vi "Dashboard Main.vi"() -> ()   [LabVIEW 2012]
uses:
  <vilib>/event_ctls.llb/eventvkey.ctl
  <vilib>/Utility/miscctls.llb/LVPointTypeDef.ctl
  <vilib>/Utility/config.llb/Read Key (String).vi
  <vilib>/Utility/config.llb/Read Key (I32).vi
  <vilib>/Utility/config.llb/Write Key (String).vi
  <vilib>/Utility/config.llb/Write Key (I32).vi
  <vilib>/Utility/config.llb/NI_LVConfig.lvlib
panel:
  in  "Camera Settings":T1={"Frate Rate"=30, "Compression"=30, "Size"=0} {"Frate Rate" scale=1.0..30.0; "Size" items=["640x480", "320x240", "160x120"]}
  out "Mode":T2(ring)=enum.""
  out "Camera IP":string="10.16.76.11"
  in  "Dashboard Tab":T3(tab)
  out "Shooter Good":bool
  out "Dashboard Code Verzion":string
  out "Robot Code Verzion":string
  out "Gyro":dbl
  out "Encoder Average":dbl
  out "Right Encoder":dbl
  out "Left Encoder":dbl
  out "Vision Angle":dbl
  in  "Debug Mode":bool
  out "Shooter Good":bool
  out "Shooter Speed":dbl(graph)
  out "Wheel Speed":dbl
  out "Shooter Output":dbl
  out "Shooter Speed":T4(ring)
  out "Robot IP":string="0.0.0.0"
  out "MotorSlide4":dbl(slide) scale=-1.0..1.0 scale format="%#_2e"
  out "MotorSlide3":dbl(slide) scale=-1.0..1.0 scale format="%#_2e"
  out "MotorSlide2":dbl(slide) scale=-1.0..1.0 scale format="%#_2e"
  in  "MotorName3":string="Front Left"
  in  "MotorName4":string="Front Right"
  in  "MotorName1":string="Rear Left"
  in  "MotorName2":string="Rear Right"
  out "MotorChart4":dbl(graph)
  out "MotorChart3":dbl(graph)
  out "MotorChart2":dbl(graph)
  out "MotorSlide1":dbl(slide) scale=-1.0..1.0 scale format="%#_2e"
  out "MotorChart1":dbl(graph)
  out "JS1 Z":dbl(slide) scale=-1.0..1.0 scale format="%#_2e"
  out "JS2 Z":dbl(slide) scale=-1.0..1.0 scale format="%#_2e"
  out "Joystick 1":cluster{"X":dbl, "Y":dbl}[](graph)
  out "Joystick 2":cluster{"X":dbl, "Y":dbl}[](graph)
  out "JS Buttons 1":T5
  out "JS Buttons 2":T5
  out "Battery Value":dbl(slide) scale=0.0..14.0 scale format="%#_2e"
  out "Battery":sgl(graph)
  in  "Slider":dbl(slide) scale=0.0..100.0 scale format="%#_3g"
  in  "On/Off":bool caption="Solenoid"
  in  "Test Name":u16(ring) items=["Select the test to run...", "Example Test", "-------------------------------", "List of tests is built in robot code.", "Replace with your own automated tests."]
  in  "Test Tree":string(tree)
  in  "Motor":cluster{"Value":dbl, "Enable":bool} {"Value" scale=-1.0..1.0 scale format="%#_3g"}
  out "Progress":T6 {"Test Progress" scale=0.0..100.0}
  in  "Rev/Fwd":cluster{"Forward":bool, "Reverse":bool}
  in  "Ring":u16(ring) items=["Auto", "Fixed indoor", "Fixed outdoor 1", "Fixed outdoor 2", "Fixed fluorescent 1", "Fixed fluorescent 2", "Hold current"]
  in  "Listbox":i32(listbox)
  in  "Viewer":T7(tab)
  out "Mbps":dbl format="%#.1g"
  in  "Enable":bool=TRUE
  in  "DB Camera Config":bool
  out "Mbps":bool
  out "fps":dbl format="%#.1g"
  out "Image Error Message":string="Timeout in Camera Communications"
  out "Camera Image":T8(plugin-control)
  out "Buttons 1":cluster{"1":bool, "2":bool, "3":bool}
  out "Kinect 1":cluster{"X":dbl, "Y":dbl, "Z":dbl} {"X" scale=1.0..-1.0; "Y" scale=1.0..-1.0; "Z" scale=1.0..-1.0}
  out "Buttons 2":cluster{"1":bool, "2":bool, "3":bool}
  out "Kinect 2":cluster{"X":dbl, "Y":dbl, "Z":dbl} {"X" scale=1.0..-1.0; "Y" scale=1.0..-1.0; "Z" scale=1.0..-1.0}
  out "Version":string
  out "Skeleton Picture":picture
  out "Players":i8
  out "Tree":string(tree)
  # "Old Info"
  # "Drive & Motors"
  # "Robot IP:"
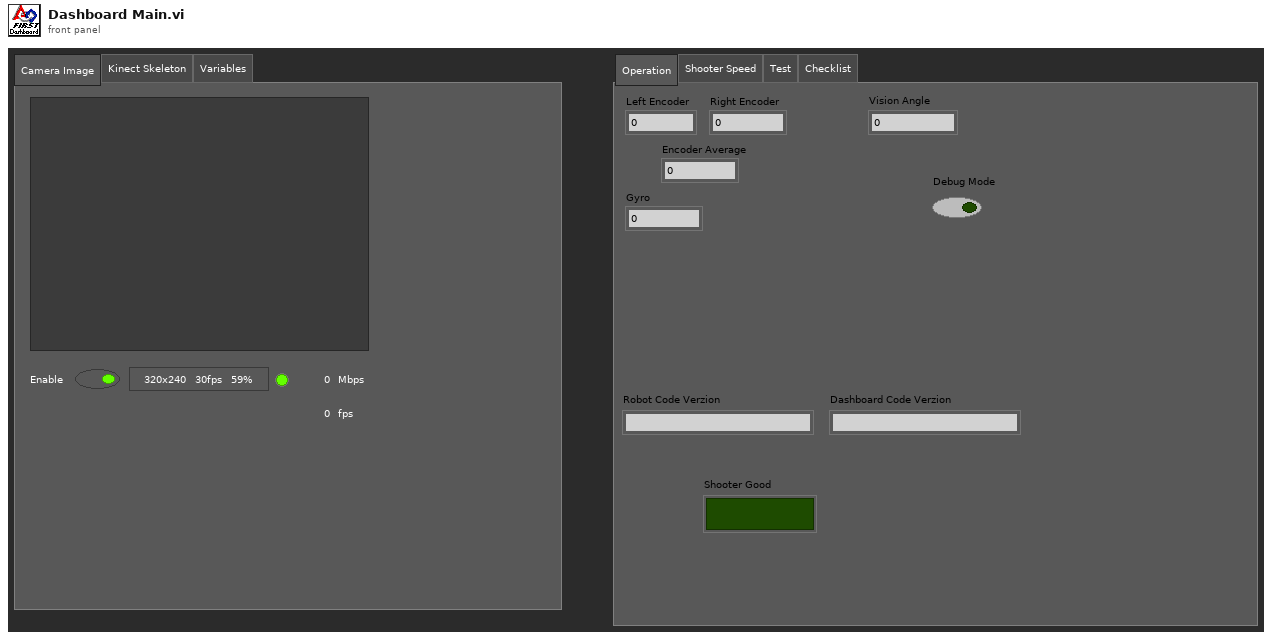
[diagram p1: front panel]
types:
  T1 = cluster{"Frate Rate":i32, "Compression":i32, "Size":u16}
  T2 = enum8{"Tele-Op Disabled", "Tele-Op Enabled", "Auto Disabled", "Auto Enabled", "Test Disabled", "Test Enabled", ""}
  T3 = enum32{"Operation", "Shooter Speed", "Test", "Checklist"}
  T4 = enum16{"Off", "Close Pyramid 3pt", "Far Pyramid 3pt", "Feeder Shot"}
  T5 = cluster{bool, bool, bool, bool, bool, bool, bool, bool, bool, bool, bool, bool}
  T6 = cluster{"Test Progress":u8, "Test Progress Text":string}
  T7 = enum32{"Camera Image", "Kinect Skeleton", "Variables"}
  T8 = typedef "IMAQ Image.ctl" = refnum<image>
  T9 = typedef "Image Type" = u32
  T10 = cluster{"Competition mode":bool, "Robot Link":bool, "Autonomous":bool, "Enabled":bool, "E-Stop":bool, "Simulated":bool, "TestMode":bool, "Docked Window":bool}
  T11 = cluster{"Boolean Array[0]":bool, "Boolean Array[1]":bool, "Boolean Array[2]":bool, "Boolean Array[3]":bool, "Boolean Array[4]":bool, "Boolean Array[5]":bool, "Boolean Array[6]":bool, "Boolean Array[7]":bool, "Boolean Array[8]":bool, "Boolean Array[9]":bool, "Boolean Array[10]":bool, "Boolean Array[11]":bool}
  T12 = typedef "LVPointTypeDef.ctl" = cluster{"Horizontal":i16, "Vertical":i16}
  T13 = typedef "LVRectTypeDef.ctl" = cluster{"Left":i16, "Top":i16, "Right":i16, "Bottom":i16}
  T14 = typedef "LVBoundsTypeDef.ctl" = cluster{"Width":u32, "Height":u32}
  T15 = typedef "SkeletonTrackState.ctl" = enum32{"NotTracked", "PositionOnly", "Tracked"}
  T16 = cluster{"TrackingState":u8[], "Position":cluster{"x":sgl, "y":sgl, "z":sgl}, cluster{"x":sgl, "y":sgl, "z":sgl, sgl}[], "TrackState":T15}
  T17 = cluster{cluster{"ScaledToPercentRange":dbl, "ScaledToPercentRange":dbl, "ScaledToPercentRange":dbl}, cluster{bool, bool, bool}}[]
  T18 = cluster{cluster{"ScaledToPercentRange":dbl, "ScaledToPercentRange":dbl, "ScaledToPercentRange":dbl}, cluster{bool, bool, bool}}
  T19 = cluster{"ScaledToPercentRange":dbl, "ScaledToPercentRange":dbl, "ScaledToPercentRange":dbl}
  T20 = typedef "NI_LVConfig.lvlib/Config Data RefNum.ctl" = refnum<k1>
  T21 = typedef "eventvkey.ctl" = enum16{"ASCII", "Enter", "Return", "Shift", "Ctrl", "Alt", "Cmd", "Opt", "Caps", "NumLock", "Clear", "Break", "Up", "Down", "Left", "Right", "Insert", "Delete", "Home", "End", "PageUp", "PageDown", "Escape", "Help", "Pause", "ScrollLock", "F1", "F2", "F3", "F4", "F5", "F6", "F7", "F8", "F9", "F10", "F11", "F12", "F13", "F14", "F15", "F16", "F17", "F18", "F19", "F20", "F21", "F22", "F23", "F24", "Play", "VolumeUp", "VolumeDown", "Mute", "Two Byte Char"}
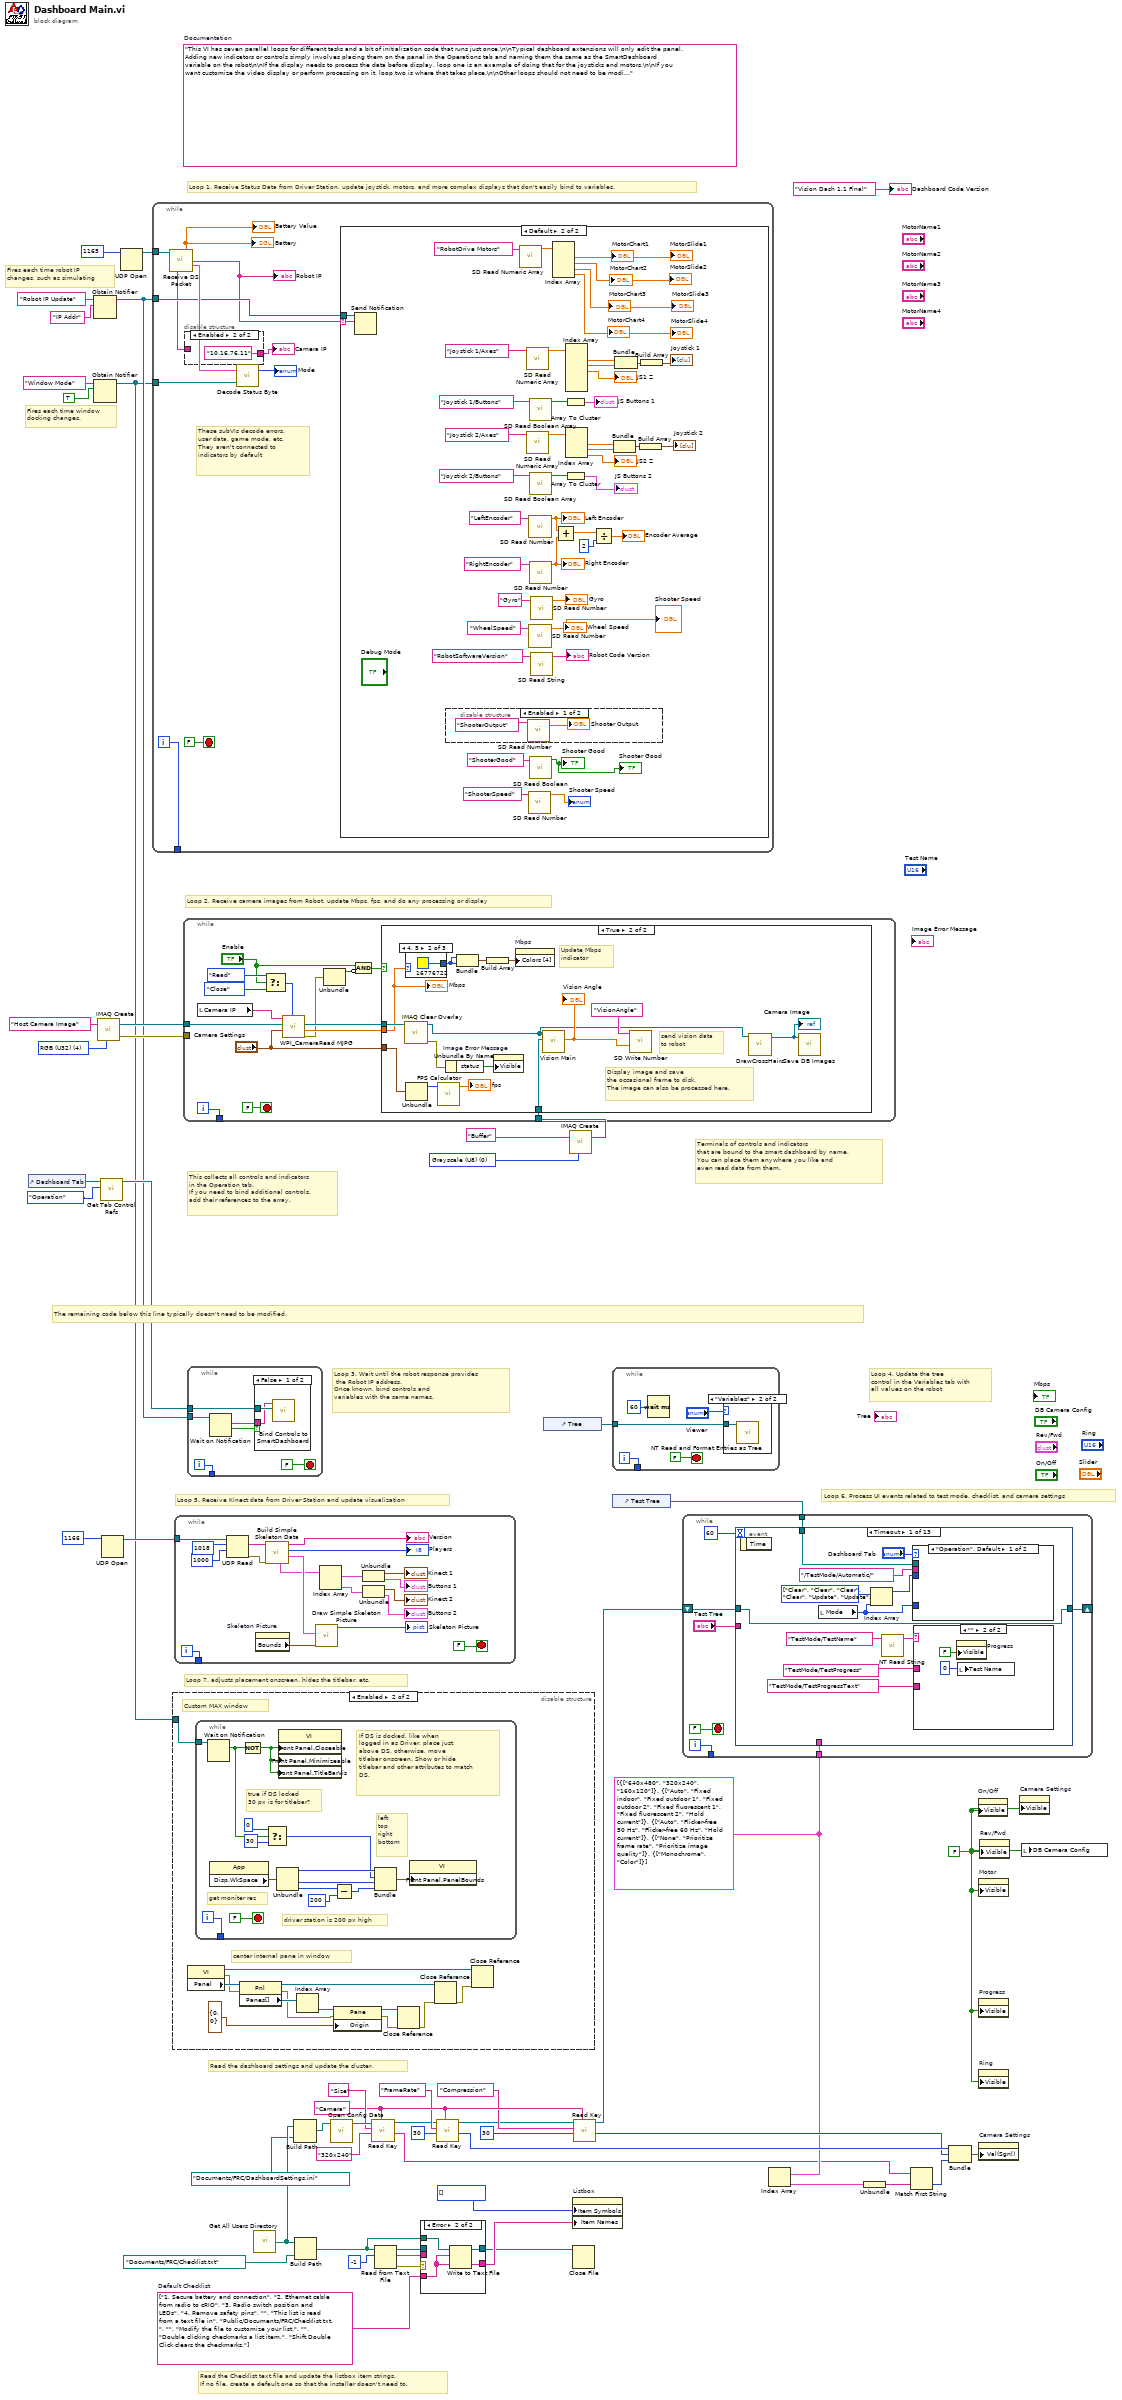
[diagram p0: block diagram]
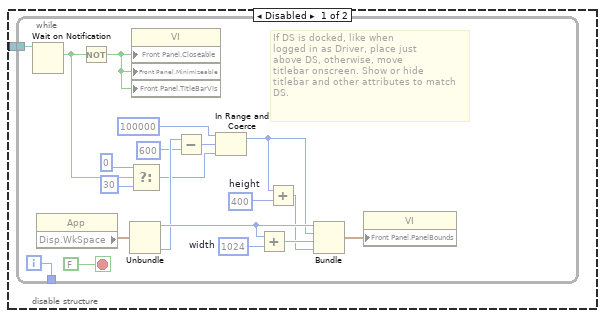
[diagram p2: hidden frame]
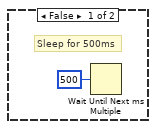
[diagram p4: hidden frame]
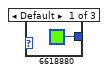
[diagram p5: hidden frame]
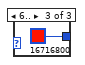
[diagram p6: hidden frame]
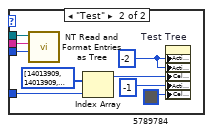
[diagram p8: hidden frame]
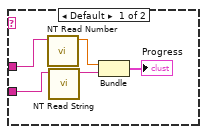
[diagram p9: hidden frame]
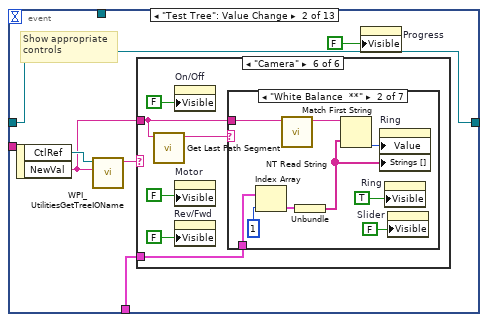
[diagram p10: hidden frame]
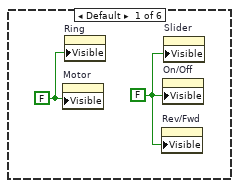
[diagram p11: hidden frame]
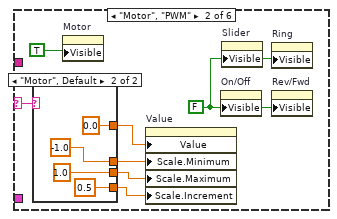
[diagram p12: hidden frame]
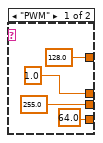
[diagram p13: hidden frame]
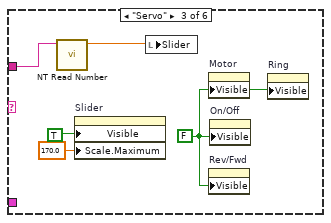
[diagram p14: hidden frame]
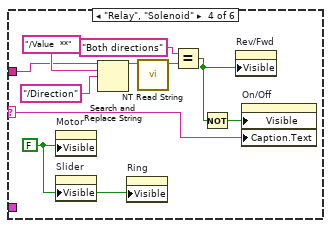
[diagram p15: hidden frame]
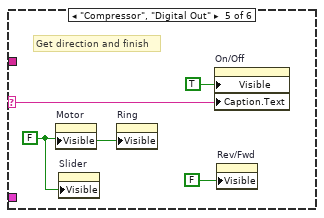
[diagram p16: hidden frame]
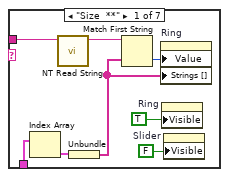
[diagram p17: hidden frame]
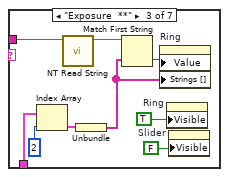
[diagram p18: hidden frame]
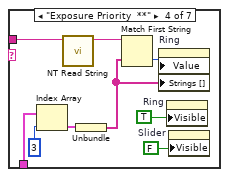
[diagram p19: hidden frame]
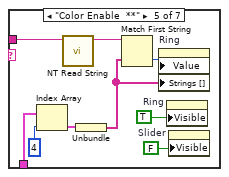
[diagram p20: hidden frame]
diagram:
  w3 = T9 0 items=["Grayscale (U8)", "Grayscale (I16)", "Grayscale (SGL)", "Complex (CSG)", "RGB (U32)", "HSL (U32)", "RGB (U64)", "Grayscale (U16)"] ("Image Type")
  w25 = "Camera"
  w17 = cluster{string[]}[] [{["640x480", "320x240", "160x120"]}, {["Auto", "Fixed indoor", "Fixed outdoor 1", "Fixed outdoor 2", "Fixed fluorescent 1", "Fixed fluorescent 2", "Hold current"]}, {["Auto", "Flicker-free 50 Hz", "Flicker-free 60 Hz", "Hold current"]}, {["None", "Prioritize frame rate", "Prioritize image quality"]}, {["Monochrome", "Color"]}]
  w33 = string[] ["1. Secure battery and connection", "2. Ethernet cable from radio to cRIO", "3. Radio switch position and LEDs", "4. Remove safety pins", "", "This list is read from a text file in", "Public/Documents/FRC/Checklist.txt.", "", "Modify the file to customize your list.", "", "Double clicking checkmarks a list item.", "Shift Double Click clears the checkmarks."]  # Default Checklist
  w31 = FALSE ("Visible")
  (unwired) "This VI has seven parallel loops for different tasks and a bit of initialization code that runs just once.\n\nTypical dashboard extensions will only edit the panel. Adding new indicators or controls simply involves placing them on the panel in the Operations tab and naming them the same as the SmartDashboard variable on the robot\n\nIf the display needs to process the data before display, loop one is an example of doing that for the joysticks and motors.\n\nIf you want customize the video display or perform processing on it, loop two is where that takes place.\n\nOther loops should not need to be modified. They are pretty standard, and document the task they perform."  # Documentation
  w54 = T9 4 items=["Grayscale (U8)", "Grayscale (I16)", "Grayscale (SGL)", "Complex (CSG)", "RGB (U32)", "HSL (U32)", "RGB (U64)"] ("Image Type")
  # "Fires each time robot IP\nchanges, such as simulating"
  # "Fires each time window\ndocking changes."
  # "Read the Checklist text file and update the listbox item strings.\nIf no file, create a default one so that the installer doesn't need to."
  # "This collects all controls and indicators\nin the Operation tab.\nIf you need to bind additional controls,\nadd their references to the array."
  # "The remaining code below this line typically doesn't need to be modified."
  # "Loop 6. Process UI events related to test mode, checklist, and camera settings"
  # "Read the dashboard settings and update the cluster."
  # "Terminals of controls and indicators\nthat are bound to the smart dashboard by name.\nYou can place them anywhere you like and\neven read data from them."
  # "Loop 4. Update the tree\ncontrol in the Variables tab with\nall values on the robot"
  # "Loop 3. Wait until the robot response provides\n the Robot IP address.\nOnce known, bind controls and\nvariables with the same names."
  # "Loop 5. Receive Kinect data from Driver Station and update visualization"
  # "Loop 7. adjusts placement onscreen, hides the titlebar, etc."
  # "Loop 1. Receive Status Data from Driver Station, update joystick, motors, and more complex displays that don't easily bind to variables."
  # "Loop 2. Receive camera images from Robot, update Mbps, fps, and do any processing or display"
  n1 = control-ref of="Dashboard Tab"() -> (w47:refnum<vi>)
  n2 = Obtain Notifier(name (unnamed)="Robot IP Update", notification data type="IP Addr" ("name (unnamed)")) -> (notifier out=w44:refnum<notifier>)  [unwired: 2 in, 2 out]
  n3 = Obtain Notifier(name (unnamed)="Window Mode", notification data type=TRUE) -> (notifier out=w37:refnum<notifier>)  [unwired: 2 in, 2 out]
  n4 = call "IMAQ Create"("Image Name"="Host Camera Image", "Image Type"=w54) -> ("New Image"=w52:T8, "error out"=w51:errorcluster)  [unwired: 2 in, 1 out]
  n5 = call <vilib>:"Get Tab Control Refs.vi"("Page Index"=enum32{"Operation", "Test"}."Operation" ("Dashboard Tab"), "TabControl in"=w47) -> ("ControlsOnPage"=w48:refnum<vi>[])  [unwired: 9 in]
  n6 = UDP Open(11:u16 1166 ("port")) -> (port=w49:refnum<k16>)  [unwired: 2 in, 4 out]
  n7 = UDP Open(11:u16 1165 ("port")) -> (port=w55:refnum<k16>)  [unwired: 2 in, 4 out]
  n8 = while {
    tunnel: w55 -> [w65]
    tunnel: w44 -> [w60]
    tunnel: w37 -> [w63]
    tunnel: [w61] -> _
    i -> [w61]
    stop <- FALSE stop-if-true
    # "These subVIs decode errors, user data, game mode, etc.\nThey aren't connected to indicators by default"
    n9 = call "Receive DS Packet.vi"("Recv Socket"=w65) -> ("Battery"=→"Battery" →"Battery Value":sgl, "Robot IP Address"=w59:string, "Status"=w66:T10, "Camera IP Address"=w57:string)  [unwired: 1 in, 10 out]
    "Robot IP" <- w59
    n10 = disable-structure shown="Enabled" {
      disable-tunnel: [w68 "10.16.76.11" ("Camera IP")] -> w58
      disable-tunnel: w57 -> [w68 _]
      frame Disabled {
      }
      frame Enabled {
      }
    }
    "Camera IP" <- w58
    n11 = call "Decode Status Byte.vi"("Window Mode Notifier"=w63, "Status"=w66) -> ("Mode"=→"Mode":T2)  [unwired: 1 out]
    n12 = case shown="Default" w59 {
      selector: w59 -> [_ w87]
      tunnel: w60 -> [_ w88]
      frame "0.0.0.0" {
        # "Robot not responding, don't poll the variables"
      }
      frame Default {
        n13 = Send Notification(notification=w87, notifier=w88) -> ()  [unwired: 1 in, 2 out]
        n14 = disable-structure shown="Enabled" {
          frame Enabled {
            n15 = call <vilib>:"SD Read Number.vi"("Name"="ShooterOutput") -> ("Numeric"=→"Shooter Output":dbl)  [unwired: 8 in, 2 out]
          }
          frame Disabled {
          }
        }
        n16 = call <vilib>:"SD Read Numeric Array.vi"("Name"="RobotDrive Motors") -> ("Numeric Array"=w111:dbl[])  [unwired: 8 in, 2 out]
        n17 = call <vilib>:"SD Read Numeric Array.vi"("Name"="Joystick 1/Axes") -> ("Numeric Array"=w104:dbl[])  [unwired: 8 in, 2 out]
        n18 = call <vilib>:"SD Read Numeric Array.vi"("Name"="Joystick 2/Axes") -> ("Numeric Array"=w98:dbl[])  [unwired: 8 in, 2 out]
        n19 = call <vilib>:"SD Read Number.vi"("Name"="ShooterSpeed") -> ("Numeric"=→"Shooter Speed":dbl)  [unwired: 8 in, 2 out]
        n20 = call <vilib>:"SD Read Number.vi"("Name"="LeftEncoder") -> ("Numeric"=w83:dbl)  [unwired: 8 in, 2 out]
        "Left Encoder" <- w83
        n21 = call <vilib>:"SD Read Number.vi"("Name"="WheelSpeed") -> ("Numeric"=→"Wheel Speed" →"Shooter Speed":dbl)  [unwired: 8 in, 2 out]
        n22 = call <vilib>:"SD Read Boolean Array.vi"("Name"="Joystick 1/Buttons") -> ("Boolean Array"=w106:bool[])  [unwired: 8 in, 2 out]
        n23 = call <vilib>:"SD Read Boolean Array.vi"("Name"="Joystick 2/Buttons") -> ("Boolean Array"=w97:bool[])  [unwired: 8 in, 2 out]
        n24 = call <vilib>:"SD Read Number.vi"("Name"="RightEncoder") -> ("Numeric"=w82:dbl)  [unwired: 8 in, 2 out]
        "Right Encoder" <- w82
        n25 = call <vilib>:"SD Read Boolean.vi"("Name"="ShooterGood") -> ("Boolean"=→"Shooter Good" →"Shooter Good":bool)  [unwired: 8 in, 2 out]
        n26 = call <vilib>:"SD Read Number.vi"("Name"="Gyro") -> ("Numeric"=→"Gyro":dbl)  [unwired: 8 in, 2 out]
        n27 = call <vilib>:"SD Read String.vi"("Name"="RobotSoftwareVersion") -> ("String"=→"Robot Code Verzion":string)  [unwired: 8 in, 2 out]
        n28 = Index Array(array=w111) -> (element #1=→"MotorChart1" →"MotorSlide1":dbl, element #2=→"MotorSlide2" →"MotorChart2":dbl, element #3=→"MotorChart3" →"MotorSlide3":dbl, element #4=→"MotorChart4" →"MotorSlide4":dbl)  [unwired: 4 in]
        n29 = Add(x=w83, y=w82) -> (x+y=w80:dbl)
        n30 = Array To Cluster(array=w106) -> (cluster=→"JS Buttons 1":T11)
        n31 = Array To Cluster(array=w97) -> (cluster=→"JS Buttons 2":T11)
        n32 = Index Array(array=w104) -> (element #1=w101:dbl, element #2=w102:dbl, element #3=→"JS1 Z":dbl)  [unwired: 6 in, 3 out]
        n33 = Index Array(array=w98) -> (element #1=w93:dbl, element #2=w92:dbl, element #3=→"JS2 Z":dbl)  [unwired: 3 in]
        n34 = Divide(x=w80, y=2) -> (x/y=→"Encoder Average":dbl)
        n35 = Bundle("Numeric"=w93, "Numeric"=w92) -> (w94:cluster{"Numeric":dbl, "Numeric":dbl})  [unwired: 1 in]
        n36 = Bundle("Numeric"=w101, "Numeric"=w102) -> (w100:cluster{"Numeric":dbl, "Numeric":dbl})  [unwired: 1 in]
        n37 = Build Array(w94) -> (→"Joystick 2":cluster{"Numeric":dbl, "Numeric":dbl}[])
        n38 = Build Array(w100) -> (→"Joystick 1":cluster{"Numeric":dbl, "Numeric":dbl}[])
      }
    }
  }
  n39 = disable-structure shown="Enabled" {
    disable-tunnel: w37 -> [w117 w150]
    frame Disabled {
      n40 = while {
        tunnel: w117 -> [w136]
        tunnel: [w134] -> _
        i -> [w134]
        stop <- FALSE stop-if-true
        w126 = 1024  # width
        w129 = 400  # height
        # "If DS is docked, like when\nlogged in as Driver, place just\nabove DS, otherwise, move\ntitlebar onscreen. Show or hide\ntitlebar and other attributes to match\nDS."
        n41 = Wait on Notification(notifier=w136) -> (notification=w121:bool)  [unwired: 3 in, 3 out]
        n42 = property class="App"() -> ("Disp.WkSpace"=w132:T13)  [unwired: 2 in, 2 out]
        n43 = Not(x=w121) -> (.not. x?=w135:bool)
        n44 = Unbundle(w132) -> ("Left"=w130:i16, "Bottom"=w127:i16)  [unwired: 2 out]
        n45 = Select(t=0, s=w121, f=30) -> (s? t:f=w120:i32)
        n46 = property class="VI"("Front Panel.Closeable"=w135, "Front Panel.Minimizeable"=w135, "Front Panel.TitleBarVis"=w135) -> ()  [unwired: 2 in, 2 out]
        n47 = Subtract(x=w127, y=600) -> (x-y=w124:i32)
        n48 = In Range and Coerce(upper limit=100000, x=w124, lower limit=w120) -> (coerced(x)=w118:i32)  [unwired: 1 out]
        n49 = Add(x=w130, y=w126) -> (x+y=w131:i32)
        n50 = Add(x=w118, y=w129) -> (x+y=w128:i32)
        n51 = Bundle("Left"=w130, w118, w131, w128) -> (w133:cluster{"Left":i16, i32, i32, i32})  [unwired: 1 out]
        n52 = property class="VI"("Front Panel.PanelBounds"=w133) -> ()  [unwired: 2 in, 2 out]
      }
    }
    frame Enabled {
      # "center internal pane in window"
      # "Custom MAX window"
      n53 = property class="VI"() -> (reference out=w143:refnum<vi>, error out=w142:errorcluster, "Panel"=w149:refnum<vi>)  [unwired: 2 in]
      n54 = while {
        tunnel: w150 -> [w164]
        tunnel: [w162] -> _
        i -> [w162]
        stop <- FALSE stop-if-true
        # "driver station is 200 px high"
        # "true if DS locked\n30 px is for titlebar?"
        # "left\ntop\nright\nbottom"
        # "get moniter rez"
        # "If DS is docked, like when\nlogged in as Driver, place just\nabove DS, otherwise, move\ntitlebar onscreen. Show or hide\ntitlebar and other attributes to match\nDS."
        n55 = Wait on Notification(notifier=w164) -> (notification=w156:bool)  [unwired: 3 in, 3 out]
        n56 = property class="App"() -> ("Disp.WkSpace"=w160:T13)  [unwired: 2 in, 2 out]
        n57 = Not(x=w156) -> (.not. x?=w163:bool)
        n58 = Select(t=0, s=w156, f=30) -> (s? t:f=w154:i32)
        n59 = Unbundle(w160) -> ("Left"=w159:i16, "Right"=w155:i16, "Bottom"=w152:i16)  [unwired: 1 out]
        n60 = property class="VI"("Front Panel.Closeable"=w163, "Front Panel.Minimizeable"=w163, "Front Panel.TitleBarVis"=w163) -> ()  [unwired: 2 in, 2 out]
        n61 = Subtract(x=w152, y=i16 200) -> (x-y=w153:i16)
        n62 = Bundle("Left"=w159, w154, "Right"=w155, w153) -> (w161:cluster{"Left":i16, i32, "Right":i16, i16})  [unwired: 1 out]
        n63 = property class="VI"("Front Panel.PanelBounds"=w161) -> ()  [unwired: 2 in, 2 out]
      }
      n64 = property class="Pnl"(reference=w149, error in=w142) -> (reference out=w144:refnum<vi>, error out=w141:errorcluster, "Panes[]"=w148:refnum<vi>[])
      n65 = Index Array(array=w148) -> (element=w147:refnum<vi>)  [unwired: 1 in]
      n66 = property class="Pane"(reference=w147, error in=w141, "Origin"=T12 {"Horizontal"=0, "Vertical"=0}) -> (reference out=w145:refnum<vi>, error out=w140:errorcluster)
      n67 = Close Reference(reference=w145, error in (no error)=w140) -> (error out=w139:errorcluster)
      n68 = Close Reference(reference=w144, error in (no error)=w139) -> (error out=w138:errorcluster)
      n69 = Close Reference(reference=w143, error in (no error)=w138) -> ()  [unwired: 1 out]
    }
  }
  n70 = while {
    tunnel: w49 -> [w182]
    tunnel: [w167] -> _
    i -> [w167]
    stop <- FALSE stop-if-true
    n71 = UDP Read(connection ID=w182, max size (548)=1018 ("bytes to read"), timeout ms (25000)=1000) -> (data out=w176:string, error out=w166:errorcluster)  [unwired: 1 in, 3 out]
    n72 = property on="Skeleton Picture" class="Pict"() -> ("Bounds"=w178:T14)  [unwired: 2 in, 2 out]
    n73 = call "Build Simple Skeleton Data.vi"("error in (no error)"=w166, "data in"=w176) -> ("Skeleton Data"=w177:T16, "NumPlayers"=→"Players":i8, "Version String"=→"Version":string, "Simple Joystick Info"=w174:T17)  [unwired: 5 in, 1 out]
    n74 = call "Draw Simple Skeleton Picture.vi"("Bounds"=w178, "Simple Skeleton"=w177) -> ("new picture out"=→"Skeleton Picture":picture)  [unwired: 9 in]
    n75 = Index Array(array=w174) -> (element #1=w173:T18, element #2=w172:T18)  [unwired: 2 in]
    n76 = Unbundle(w173) -> (→"Kinect 1":T19, →"Buttons 1":cluster{bool, bool, bool})
    n77 = Unbundle(w172) -> (→"Kinect 2":T19, →"Buttons 2":cluster{bool, bool, bool})
  }
  n78 = while {
    tunnel: w48 -> [w190]
    tunnel: w44 -> [w187]
    tunnel: [w185] -> _
    i -> [w185]
    stop <- FALSE stop-if-true
    n79 = Wait on Notification(notifier=w187) -> (notification=w186:string, timed out?=w188:bool)  [unwired: 3 in, 2 out]
    n80 = case shown="False" w188 {
      tunnel: w190 -> [w192 _]
      tunnel: w186 -> [w191 _]
      frame False {
        n81 = call <vilib>:"Bind Controls to SmartDashboard.vi"("Bound Control Refs"=w192, "Server IP Address"=w191) -> ()  [unwired: 10 in]
      }
      frame True {
      }
    }
  }
  n82 = call "Get All Users Directory.vi"() -> ("All User Path"=w30:path)
  n83 = Build Path(base path=w30, name or relative path=path "Documents/FRC/DashboardSettings.ini") -> (appended path=w29:path)
  n84 = Build Path(base path=w30, name or relative path=path "Documents/FRC/Checklist.txt") -> (appended path=w34:path)
  n85 = call <vilib>:"Open Config Data.vi"("configuration file path"=w29) -> ("refnum"=w28:T20)  [unwired: 8 in, 2 out]
  n86 = call-poly <vilib>:"Read Key.vi"("section"=w25, "default value"="320x240", "key"="Size", "refnum"=w28) -> ("value"=w15:string, "refnum out"=w10:T20)  [unwired: 2 in, 4 out]
  n87 = Read from Text File(file (use dialog)=w34, count=-1 ("timeout ms (25000)")) -> (refnum out=w12:refnum<file>, text=w35:string[], error out=w36:errorcluster)  [unwired: 2 in, 1 out]
  n88 = case shown="Error" w36 {
    tunnel: w35 -> [w194 _]
    tunnel: [w194 w196] -> w32
    tunnel: w33 -> [_ w196]
    tunnel: w34 -> [_ w197]
    tunnel: [w193 w195] -> w11
    tunnel: w12 -> [w193 _]
    frame No Error {
    }
    frame Error {
      n89 = Write to Text File(file (use dialog)=w197, text=w196) -> (refnum out=w195:refnum<file>)  [unwired: 2 in, 2 out]
    }
  }
  n90 = call-poly <vilib>:"Read Key.vi"("section"=w25, "default value"=30, "key"="FrameRate", "refnum"=w10) -> ("value"=w20:i32, "refnum out"=w9:T20)  [unwired: 1 in, 5 out]
  n91 = control-ref of="Tree"() -> (w6:refnum<vi>)
  n92 = call "IMAQ Create"("Image Name"="Buffer", "Image Type"=w3) -> ("New Image"=w2:T8)  [unwired: 3 in, 1 out]
  n93 = while {
    tunnel: w52 -> [w208]
    tunnel: w51 -> [_]
    tunnel: [w211] -> _
    tunnel: w2 -> [w198]
    i -> [w211]
    stop <- FALSE stop-if-true
    n94 = local read "Camera IP"() -> (w210:string)
    n95 = Select(t=enum16{"Read", "Reopen", "Close"}."Read" ("Operation"), s="Enable", f=enum16{"Read", "Reopen", "Close"}."Close" ("Operation")) -> (s? t:f=w203:enum16{"Read", "Reopen", "Close"})
    n96 = call <vilib>:"WPI_CameraRead MJPG.vi"("Operation"=w203, "Camera Settings"="Camera Settings", "Image"=w208, "address"=w210) -> ("error out"=w202:errorcluster, "Bandwidth (kbps)"=w206:dbl, "Image Out"=w207:T8)  [unwired: 5 in]
    n97 = Unbundle(w202) -> ("status"=w200:bool)  [unwired: 2 out]
    n98 = Compound Arithmetic op=AND("Enable", invert w200) -> (w199:bool)
    n99 = case shown="True" w199 {
      tunnel: "Camera Settings" -> [_ w220]
      tunnel: w207 -> [_ w223]
      tunnel: w206 -> [_ w222]
      tunnel: w198 -> [_ w218]
      frame False {
        # "Sleep for 500ms"
        n100 = Wait Until Next ms Multiple(millisecond multiple=u32 500) -> ()  [unwired: 1 out]
      }
      frame True {
        # "send vision data\nto robot"
        # "Display image and save\nthe occasional frame to disk.\nThe image can also be processed here."
        # "Update Mbps\nindicator"
        n101 = call "IMAQ Clear Overlay"("Image"=w223) -> ("error out"=w227:errorcluster, "Image Out"=w214:T8)  [unwired: 2 in, 7 out]
        n102 = case shown="4, 5" w222 {
          tunnel: [u32 6618880 ("Color Box") u32 16776722 ("Color Box") u32 16716800 ("Color Box")] -> w224
          frame Default {
          }
          frame 4, 5 {
          }
          frame 6.. {
          }
        }
        n103 = Unbundle(w220) -> ("Frate Rate"=w219:i32)  [unwired: 2 out]
        n104 = call "FPS Calculator.vi"("Average Count"=w219) -> ("fps"=→"fps":dbl)  [unwired: 10 in]
        n105 = Unbundle By Name(w227) -> ("status"=w228:bool)
        n106 = Bundle("Color Box"=w224, "Color Box"=w224) -> (w226:cluster{"Color Box":u32, "Color Box":u32})  [unwired: 1 out]
        n107 = Build Array(w226) -> (w225:cluster{"Color Box":u32, "Color Box":u32}[])
        n108 = property on="Image Error Message" class="Str"("Visible"=w228) -> ()  [unwired: 2 in, 2 out]
        n109 = property on="Mbps" class="Bool (strict)"("Colors [4]"=w225) -> ()  [unwired: 2 in, 2 out]
        n110 = call "Vision Main.vi"("Frame Buffer"=w218, "Camera Image"=w214) -> ("Chosen Target Angle"=w216:dbl)  [unwired: 8 in, 1 out]
        "Vision Angle" <- w216
        n111 = call <vilib>:"SD Write Number.vi"("Numeric"=w216, "Name"="VisionAngle") -> ()  [unwired: 8 in, 2 out]
        n112 = call "DrawCrossHairs.vi"("Image In"=w214) -> ("Image Out"=w215:T8)  [unwired: 10 in]
        "Camera Image" <- w215
        n113 = call "Save DB Images.vi"("Image"=w215) -> ()  [unwired: 2 in, 1 out]
        "Mbps" <- w222
      }
    }
  }
  n114 = property on="Listbox" class="LstBox (strict)"("Item Symbols"=i32[] [], "Item Names"=w32) -> ()  [unwired: 2 in, 2 out]
  n115 = Close File(refnum=w11) -> ()  [unwired: 1 in, 2 out]
  n116 = call-poly <vilib>:"Read Key.vi"("section"=w25, "default value"=30, "key"="Compression", "refnum"=w9) -> ("value"=w19:i32, "refnum out"=w7:T20)  [unwired: 1 in, 5 out]
  n117 = while {
    tunnel: [w233] -> _
    tunnel: w6 -> [w232]
    i -> [w233]
    stop <- FALSE stop-if-true
    n118 = Wait (ms)(milliseconds to wait=u32 60) -> ()  [unwired: 1 out]
    n119 = case shown="\"Variables\"" "Viewer" {
      tunnel: w232 -> [_ w237]
      frame Default {
      }
      frame "Variables" {
        n120 = call <vilib>:"NT Read and Format Entries as Tree.vi"("Tree Refnum"=w237) -> ()  [unwired: 9 in, 2 out]
      }
    }
  }
  n121 = control-ref of="Test Tree"() -> (w5:refnum<vi>)
  n122 = while {
    tunnel: w17 -> [w242]
    shift-right: [w241] -> _
    shift-left: w7 -> [w240]
    tunnel: [w239] -> _
    tunnel: w5 -> [w238]
    i -> [w239]
    stop <- FALSE stop-if-true
    n123 = event shown="[0] Timeout" {
      selector: _ -> [_ _ _ _ _ _ _ _ _ _ _ _ _]
      dyn-events: _ -> [_ _ _ _ _ _ _ _ _ _ _ _ _]
      timeout: u32 60 ("milliseconds to wait") -> [_ _ _ _ _ _ _ _ _ _ _ _ _]
      tunnel: w238 -> [w252 _ _ _ _ _ _ _ _ _ _ _ _]
      tunnel: "Test Tree" -> [_ _ _ _ _ _ _ _ w446 w454 w456 w460 w468]
      tunnel: w242 -> [_ w274 _ _ _ _ w410 w440 _ _ _ _ _]
      tunnel: [w246 w273 _ w376 w384 w396 w409 w433 w445 w452 w455 w459 w467] -> w241
      tunnel: w240 -> [w246 w273 _ w376 w384 w396 w408 w433 w445 w452 w455 w459 w467]
      event Timeout {
        w251 = enum16{"Update", "Clear"}[] [enum."Clear", enum."Clear", enum."Clear", enum."Clear", enum."Update", enum."Update", enum."Clear"] items=["Update", "Clear"]
        n124 = event-data() -> ()  [unwired: 1 in, 1 out]
        n125 = local read "Mode"() -> (w249:T2)
        n126 = Index Array(array=w251, index=w249) -> (element=w250:enum16{"Update", "Clear"})
        n127 = call <vilib>:"NT Read String.vi"("Name"="TestMode/TestName") -> ("String"=w255:string)  [unwired: 9 in, 1 out]
        n128 = case shown="\"Operation\", Default" "Dashboard Tab" {
          tunnel: w252 -> [_ w265]
          tunnel: "/TestMode/Automatic/" ("Name Pattern") -> [_ w264]
          tunnel: w250 -> [_ w263]
          tunnel: w249 -> [_ w261]
          frame "Operation", Default {
          }
          frame "Test" {
            w260 = -2 ("Active Item:Row Number")
            n129 = call <vilib>:"NT Read and Format Entries as Tree.vi"("Operation"=w263, "Name Pattern"=w264, "Tree Refnum"=w265) -> ()  [unwired: 7 in, 2 out]
            n130 = Index Array(array=u32[] [14013909, 14013909, 14013909, 14013909, 14013909, 16777215, 14013909], index=w261) -> (element=w259:u32)
            n131 = property on="Test Tree" class="Tree (strict)"("Active Item Row Number"=w260, "ActiveColNum"=w260, "CellBG"=w259, "Active Item Row Number"=-1 ("Active Item:Row Number"), "CellBG"=u32 5789784 ("Color Box")) -> ()  [unwired: 2 in, 2 out]
          }
        }
        n132 = case shown="\"\"" w255 {
          tunnel: "TestMode/TestProgress" ("Name") -> [w267 _]
          tunnel: "TestMode/TestProgressText" ("Name") -> [w266 _]
          frame Default {
            n133 = call <vilib>:"NT Read Number.vi"("Name"=w267) -> ("Numeric"=w268:dbl)  [unwired: 9 in, 1 out]
            n134 = call <vilib>:"NT Read String.vi"("Name"=w266) -> ("String"=w269:string)  [unwired: 9 in, 1 out]
            n135 = Bundle("Numeric"=w268, "String"=w269) -> (→"Progress":cluster{"Numeric":dbl, "String":string})  [unwired: 1 in]
          }
          frame "" {
            n136 = property on="Progress" class="Clust (strict)"("Visible"=FALSE) -> ()  [unwired: 2 in, 2 out]
            n137 = local write "Test Name"(u16 0) -> ()
          }
        }
      }
      event "Test Tree": Value Change {
        # "Show appropriate\ncontrols"
        n138 = event-data() -> ("CtlRef"=w277:refnum<vi>, "NewVal"=w275:string)  [unwired: 1 in]
        n139 = call <vilib>:"WPI_UtilitiesGetTreeIOName.vi"("NewVal"=w275, "TreeControl in"=w277) -> ("I/O Name"=w278:string)  [unwired: 9 in]
        n140 = case shown="\"Camera\"" w278 {
          selector: w278 -> [_ w285 _ w303 w312 _]
          tunnel: w275 -> [_ _ w300 w302 _ w319]
          tunnel: w274 -> [_ _ _ _ _ w318]
          frame Default {
            w280 = FALSE ("Visible")
            w279 = FALSE ("Visible")
            n141 = property on="Motor" class="Clust (strict)"("Visible"=w279) -> ()  [unwired: 2 in, 2 out]
            n142 = property on="Ring" class="Ring (strict)"("Visible"=w279) -> ()  [unwired: 2 in, 2 out]
            n143 = property on="Rev/Fwd" class="Clust (strict)"("Visible"=w280) -> ()  [unwired: 2 in, 2 out]
            n144 = property on="On/Off" class="Bool (strict)"("Visible"=w280) -> ()  [unwired: 2 in, 2 out]
            n145 = property on="Slider" class="Slide (strict)"("Visible"=w280) -> ()  [unwired: 2 in, 2 out]
          }
          frame "Motor", "PWM" {
            w286 = FALSE ("Visible")
            n146 = case shown="\"Motor\", Default" w285 {
              tunnel: [1.0 ("Value") -1.0 ("Value")] -> w284
              tunnel: [255.0 ("Value") 1.0 ("Value")] -> w283
              tunnel: [128.0 ("Value") 0.0 ("Value")] -> w282
              tunnel: [64.0 ("Value") 0.5 ("Value")] -> w281
              frame "PWM" {
              }
              frame "Motor", Default {
              }
            }
            n147 = property on="Motor" class="Clust (strict)"("Visible"=TRUE) -> ()  [unwired: 2 in, 2 out]
            n148 = property on="Value" class="Slide (strict)"("Value"=w282, "Scale.Minimum"=w284, "Scale.Maximum"=w283, "Scale.Increment"=w281) -> ()  [unwired: 2 in, 2 out]
            n149 = property on="On/Off" class="Bool (strict)"("Visible"=w286) -> ()  [unwired: 2 in, 2 out]
            n150 = property on="Slider" class="Slide (strict)"("Visible"=w286) -> ()  [unwired: 2 in, 2 out]
            n151 = property on="Ring" class="Ring (strict)"("Visible"=w286) -> ()  [unwired: 2 in, 2 out]
            n152 = property on="Rev/Fwd" class="Clust (strict)"("Visible"=w286) -> ()  [unwired: 2 in, 2 out]
          }
          frame "Servo" {
            w298 = FALSE ("Visible")
            n153 = call <vilib>:"NT Read Number.vi"("Name"=w300) -> ("Numeric"=w299:dbl)  [unwired: 9 in, 1 out]
            n154 = property on="Slider" class="Slide (strict)"("Visible"=TRUE, "Scale.Maximum"=170.0 ("Scale.Range:Maximum")) -> ()  [unwired: 2 in, 2 out]
            n155 = local write "Slider"(w299) -> ()
            n156 = property on="Motor" class="Clust (strict)"("Visible"=w298) -> ()  [unwired: 2 in, 2 out]
            n157 = property on="Rev/Fwd" class="Clust (strict)"("Visible"=w298) -> ()  [unwired: 2 in, 2 out]
            n158 = property on="On/Off" class="Bool (strict)"("Visible"=w298) -> ()  [unwired: 2 in, 2 out]
            n159 = property on="Ring" class="Ring (strict)"("Visible"=w298) -> ()  [unwired: 2 in, 2 out]
          }
          frame "Relay", "Solenoid" {
            w301 = FALSE ("Visible")
            n160 = property on="Motor" class="Clust (strict)"("Visible"=w301) -> ()  [unwired: 2 in, 2 out]
            n161 = property on="Slider" class="Slide (strict)"("Visible"=w301) -> ()  [unwired: 2 in, 2 out]
            n162 = Search and Replace String(input string=w302, search string="/Value  **", replace string="/Direction") -> (result string=w308:string)  [unwired: 5 in, 3 out]
            n163 = property on="Ring" class="Ring (strict)"("Visible"=w301) -> ()  [unwired: 2 in, 2 out]
            n164 = call <vilib>:"NT Read String.vi"("Name"=w308) -> ("String"=w306:string)  [unwired: 9 in, 1 out]
            n165 = Equal?(x="Both directions", y=w306) -> (x = y?=w304:bool)
            n166 = Not(x=w304) -> (.not. x?=w305:bool)
            n167 = property on="Rev/Fwd" class="Clust (strict)"("Visible"=w304) -> ()  [unwired: 2 in, 2 out]
            n168 = property on="On/Off" class="Bool (strict)"("Visible"=w305, "Caption.Text"=w303) -> ()  [unwired: 2 in, 2 out]
          }
          frame "Compressor", "Digital Out" {
            w311 = FALSE ("Visible")
            # "Get direction and finish"
            n169 = property on="Motor" class="Clust (strict)"("Visible"=w311) -> ()  [unwired: 2 in, 2 out]
            n170 = property on="Slider" class="Slide (strict)"("Visible"=w311) -> ()  [unwired: 2 in, 2 out]
            n171 = property on="Ring" class="Ring (strict)"("Visible"=w311) -> ()  [unwired: 2 in, 2 out]
            n172 = property on="On/Off" class="Bool (strict)"("Visible"=TRUE, "Caption.Text"=w312) -> ()  [unwired: 2 in, 2 out]
            n173 = property on="Rev/Fwd" class="Clust (strict)"("Visible"=FALSE) -> ()  [unwired: 2 in, 2 out]
          }
          frame "Camera" {
            n174 = call <vilib>:"Get Last Path Segment.vi"("String in"=w319) -> ("String out"=w320:string)  [unwired: 10 in]
            n175 = property on="On/Off" class="Bool (strict)"("Visible"=FALSE) -> ()  [unwired: 2 in, 2 out]
            n176 = property on="Motor" class="Clust (strict)"("Visible"=FALSE) -> ()  [unwired: 2 in, 2 out]
            n177 = property on="Rev/Fwd" class="Clust (strict)"("Visible"=FALSE) -> ()  [unwired: 2 in, 2 out]
            n178 = case shown="\"White Balance  **\"" w320 {
              tunnel: w319 -> [w326 w335 w344 w353 w362 _ w368]
              tunnel: w318 -> [w324 w332 w341 w350 w359 _ _]
              frame "Size  **" {
                n179 = Index Array(array=w324) -> (element=w323:cluster{string[]})  [unwired: 1 in]
                n180 = call <vilib>:"NT Read String.vi"("Name"=w326) -> ("String"=w325:string)  [unwired: 9 in, 1 out]
                n181 = Unbundle(w323) -> (w321:string[])
                n182 = Match First String(2:w321, 3:w325) -> (0:w322:i32)  [unwired: 1 out]
                n183 = property on="Ring" class="Ring (strict)"("Value"=w322, "Strings []"=w321) -> ()  [unwired: 2 in, 2 out]
                n184 = property on="Ring" class="Ring (strict)"("Visible"=TRUE) -> ()  [unwired: 2 in, 2 out]
                n185 = property on="Slider" class="Slide (strict)"("Visible"=FALSE) -> ()  [unwired: 2 in, 2 out]
              }
              frame "White Balance  **" {
                n186 = Index Array(array=w332, index=1) -> (element=w333:cluster{string[]})
                n187 = call <vilib>:"NT Read String.vi"("Name"=w335) -> ("String"=w334:string)  [unwired: 9 in, 1 out]
                n188 = Unbundle(w333) -> (w330:string[])
                n189 = Match First String(2:w330, 3:w334) -> (0:w329:i32)  [unwired: 1 out]
                n190 = property on="Ring" class="Ring (strict)"("Value"=w329, "Strings []"=w330) -> ()  [unwired: 2 in, 2 out]
                n191 = property on="Ring" class="Ring (strict)"("Visible"=TRUE) -> ()  [unwired: 2 in, 2 out]
                n192 = property on="Slider" class="Slide (strict)"("Visible"=FALSE) -> ()  [unwired: 2 in, 2 out]
              }
              frame "Exposure  **" {
                n193 = Index Array(array=w341, index=2) -> (element=w342:cluster{string[]})
                n194 = call <vilib>:"NT Read String.vi"("Name"=w344) -> ("String"=w343:string)  [unwired: 9 in, 1 out]
                n195 = Unbundle(w342) -> (w338:string[])
                n196 = Match First String(2:w338, 3:w343) -> (0:w339:i32)  [unwired: 1 out]
                n197 = property on="Ring" class="Ring (strict)"("Value"=w339, "Strings []"=w338) -> ()  [unwired: 2 in, 2 out]
                n198 = property on="Ring" class="Ring (strict)"("Visible"=TRUE) -> ()  [unwired: 2 in, 2 out]
                n199 = property on="Slider" class="Slide (strict)"("Visible"=FALSE) -> ()  [unwired: 2 in, 2 out]
              }
              frame "Exposure Priority  **" {
                n200 = Index Array(array=w350, index=3) -> (element=w351:cluster{string[]})
                n201 = call <vilib>:"NT Read String.vi"("Name"=w353) -> ("String"=w352:string)  [unwired: 9 in, 1 out]
                n202 = Unbundle(w351) -> (w347:string[])
                n203 = Match First String(2:w347, 3:w352) -> (0:w348:i32)  [unwired: 1 out]
                n204 = property on="Ring" class="Ring (strict)"("Value"=w348, "Strings []"=w347) -> ()  [unwired: 2 in, 2 out]
                n205 = property on="Ring" class="Ring (strict)"("Visible"=TRUE) -> ()  [unwired: 2 in, 2 out]
                n206 = property on="Slider" class="Slide (strict)"("Visible"=FALSE) -> ()  [unwired: 2 in, 2 out]
              }
              frame "Color Enable  **" {
                n207 = Index Array(array=w359, index=4) -> (element=w360:cluster{string[]})
                n208 = call <vilib>:"NT Read String.vi"("Name"=w362) -> ("String"=w361:string)  [unwired: 9 in, 1 out]
                n209 = Unbundle(w360) -> (w356:string[])
                n210 = Match First String(2:w356, 3:w361) -> (0:w357:i32)  [unwired: 1 out]
                n211 = property on="Ring" class="Ring (strict)"("Value"=w357, "Strings []"=w356) -> ()  [unwired: 2 in, 2 out]
                n212 = property on="Ring" class="Ring (strict)"("Visible"=TRUE) -> ()  [unwired: 2 in, 2 out]
                n213 = property on="Slider" class="Slide (strict)"("Visible"=FALSE) -> ()  [unwired: 2 in, 2 out]
              }
              frame Default {
                n214 = property on="Ring" class="Ring (strict)"("Visible"=FALSE) -> ()  [unwired: 2 in, 2 out]
                n215 = property on="Slider" class="Slide (strict)"("Visible"=FALSE) -> ()  [unwired: 2 in, 2 out]
              }
              frame "Brightness  **", "Color Level  **", "Compression  **", "FPS  **", "Sharpness  **" {
                n216 = call <vilib>:"NT Read Number.vi"("Name"=w368) -> ("Numeric"=w367:dbl)  [unwired: 9 in, 1 out]
                n217 = local write "Slider"(w367) -> ()
                n218 = property on="Slider" class="Slide (strict)"("Visible"=TRUE, "Scale.Maximum"=100.0 ("Scale.Range:Maximum")) -> ()  [unwired: 2 in, 2 out]
                n219 = property on="Ring" class="Ring (strict)"("Visible"=FALSE) -> ()  [unwired: 2 in, 2 out]
              }
            }
          }
        }
        n220 = property on="Progress" class="Clust (strict)"("Visible"=FALSE) -> ()  [unwired: 2 in, 2 out]
      }
      event "Test Name": Mouse Enter {
        # "Populate the ring with the list of tests"
        n221 = event-data() -> ()  [unwired: 1 in, 1 out]
        n222 = call <vilib>:"NT Read String Array.vi"("Name"="TestMode/TestList") -> ("String Array"=w375:string[])  [unwired: 9 in, 1 out]
        n223 = Build Array (concatenate)("Select the test to run...", w375) -> (w374:string[])
        n224 = property on="Test Name" class="Ring (strict)"("Strings []"=w374) -> ()  [unwired: 2 in, 2 out]
      }
      event "Test Name": Value Change {
        w377 = FALSE ("Visible")
        # "Tell the robot the test name to run"
        n225 = event-data() -> ("NewVal"=w381:u16)  [unwired: 1 in]
        n226 = property on="Test Name" class="Ring (strict)"() -> ("Strings []"=w382:string[])  [unwired: 2 in, 2 out]
        n227 = local write "Progress"(T6 {"Test Progress"=0, "Test Progress Text"=""} ("Progress")) -> ()
        n228 = Index Array(array=w382, index=w381) -> (element=w380:string)
        n229 = call <vilib>:"NT Write String.vi"("String"=w380, "Name"="TestMode/TestName") -> ()  [unwired: 9 in, 1 out]
        n230 = property on="Progress" class="Clust (strict)"("Visible"=TRUE) -> ()  [unwired: 2 in, 2 out]
        n231 = property on="Motor" class="Clust (strict)"("Visible"=w377) -> ()  [unwired: 2 in, 2 out]
        n232 = property on="Slider" class="Slide (strict)"("Visible"=w377) -> ()  [unwired: 2 in, 2 out]
        n233 = property on="On/Off" class="Bool (strict)"("Visible"=w377) -> ()  [unwired: 2 in, 2 out]
        n234 = property on="Rev/Fwd" class="Clust (strict)"("Visible"=w377) -> ()  [unwired: 2 in, 2 out]
        n235 = property on="Ring" class="Ring (strict)"("Visible"=w377) -> ()  [unwired: 2 in, 2 out]
      }
      event "Listbox": Double Click {
        n236 = event-data() -> ("PlatMods.Shift"=w385:bool, "Row"=w387:i32)  [unwired: 1 in]
        n237 = case shown="False" w385 {
          tunnel: w387 -> [w391 _]
          tunnel: 1 -> [w390 _]
          frame False {
            n238 = property on="Listbox" class="LstBox (strict)"() -> ("Item Symbols"=w389:i32[])  [unwired: 2 in, 2 out]
            n239 = Replace Array Subset(array=w389, new element=w390, index=w391) -> (w388:i32[])
            n240 = property on="Listbox" class="LstBox (strict)"("Item Symbols"=w388) -> ()  [unwired: 2 in, 2 out]
          }
          frame True {
            w392 = 0 ("Top Row")
            n241 = property on="Listbox" class="LstBox (strict)"() -> ("Number of Rows"=w394:u32)  [unwired: 2 in, 2 out]
            n242 = Initialize Array(0, w394) -> (w393:i32[])
            n243 = property on="Listbox" class="LstBox (strict)"("Top Row"=w392, "Value"=w392, "Item Symbols"=w393) -> ()  [unwired: 2 in, 2 out]
          }
        }
      }
      event "Listbox": Key Down {
        n244 = event-data() -> ("VKey"=w398:T21)  [unwired: 1 in]
        n245 = case shown="\"Left\", \"Right\"" w398 {
          selector: w398 -> [w403 _]
          tunnel: eventvkey."Left" ("VKey") -> [w401 _]
          frame "Left", "Right" {
            n246 = Equal?(x=w401, y=w403) -> (x = y?=w402:bool)
            n247 = Select(t=0, s=w402, f=1) -> (s? t:f=w404:i32)
            n248 = property on="Listbox" class="LstBox (strict)"() -> ("Item Symbols"=w407:i32[])  [unwired: 2 in, 2 out]
            n249 = Replace Array Subset(array=w407, new element=w404, index="Listbox") -> (w406:i32[])
            n250 = property on="Listbox" class="LstBox (strict)"("Item Symbols"=w406) -> ()  [unwired: 2 in, 2 out]
          }
          frame Default {
          }
        }
      }
      event "DB Camera Config": Value Change {
        n251 = event-data() -> ("NewVal"=w411:bool)  [unwired: 1 in]
        n252 = case shown="False" w411 {
          tunnel: w410 -> [w420 _]
          tunnel: [w413 w431] -> w409
          tunnel: w408 -> [w412 w431]
          frame False {
            w427 = "Camera"
            w430 = FALSE ("Visible")
            n253 = local read "Camera Settings"() -> (w419:T1)
            n254 = Index Array(array=w420) -> (element=w423:cluster{string[]})  [unwired: 1 in]
            n255 = Unbundle(w419) -> ("Frate Rate"=w418:i32, "Compression"=w417:i32, "Size"=w421:u16)
            n256 = Unbundle(w423) -> (w422:string[])
            n257 = Index Array(array=w422, index=w421) -> (element=w416:string)
            n258 = call-poly <vilib>:"Write Key.vi"("section"=w427, "value"=w416, "key"="Size", "refnum"=w412) -> ("refnum out"=w429:T20)  [unwired: 2 in, 5 out]
            n259 = call-poly <vilib>:"Write Key.vi"("section"=w427, "value"=w418, "key"="FrameRate", "refnum"=w429) -> ("refnum out"=w428:T20)  [unwired: 1 in, 6 out]
            n260 = property on="Camera Settings" class="Clust (strict)"("Visible"=w430) -> ()  [unwired: 2 in, 2 out]
            n261 = local write "DB Camera Config"(w430) -> ()
            n262 = call-poly <vilib>:"Write Key.vi"("section"=w427, "value"=w417, "key"="Compression", "refnum"=w428) -> ("refnum out"=w414:T20)  [unwired: 1 in, 6 out]
            n263 = call <vilib>:"Close Config Data.vi"("refnum"=w414) -> ("file path"=w415:path)  [unwired: 2 in, 8 out]
            n264 = call <vilib>:"Open Config Data.vi"("configuration file path"=w415) -> ("refnum"=w413:T20)  [unwired: 8 in, 2 out]
          }
          frame True {
            n265 = property on="Camera Settings" class="Clust (strict)"("Visible"=TRUE) -> ()  [unwired: 2 in, 2 out]
          }
        }
      }
      event "Camera Settings": Value Change {
        n266 = event-data() -> ("NewVal"=w444:T1)  [unwired: 1 in]
        n267 = Index Array(array=w440) -> (element=w439:cluster{string[]})  [unwired: 1 in]
        n268 = Unbundle(w444) -> ("Frate Rate"=w435:i32, "Compression"=w434:i32, "Size"=w437:u16)
        n269 = Unbundle(w439) -> (w438:string[])
        n270 = Index Array(array=w438, index=w437) -> (element=w436:string)
        n271 = Format Into String(format string="%s   %dfps   %d%%", w436, w435, w434) -> (resulting string=w441:string)  [unwired: 2 in, 1 out]
        n272 = Build Array(w441) -> (w442:string[])
        n273 = property on="DB Camera Config" class="Bool (strict)"("Strings [4]"=w442) -> ()  [unwired: 2 in, 2 out]
      }
      event "Motor.Enable": Value Change {
        n274 = event-data() -> ("NewVal"=w450:bool)  [unwired: 1 in]
        n275 = Unbundle("Motor") -> ("Value"=w449:dbl)  [unwired: 1 out]
        n276 = Select(t=w449, s=w450, f=0.0) -> (s? t:f=w447:dbl)
        n277 = call <vilib>:"NT Write Number.vi"("Numeric"=w447, "Name"=w446) -> ()  [unwired: 9 in, 1 out]
      }
      event "Slider": Value Change {
        n278 = event-data() -> ("NewVal"=w453:dbl)  [unwired: 1 in]
        n279 = call <vilib>:"NT Write Number.vi"("Numeric"=w453, "Name"=w454) -> ()  [unwired: 9 in, 1 out]
      }
      event "On/Off": Value Change {
        n280 = event-data() -> ("NewVal"=w458:bool)  [unwired: 1 in]
        n281 = Boolean To (0,1)(Boolean=w458) -> (0, 1=w457:i16)
        n282 = call <vilib>:"NT Write Number.vi"("Numeric"=w457, "Name"=w456) -> ()  [unwired: 9 in, 1 out]
      }
      event "Rev/Fwd": Value Change {
        n283 = event-data() -> ("NewVal.Forward"=w466:bool, "NewVal.Reverse"=w465:bool)  [unwired: 1 in]
        n284 = Boolean To (0,1)(Boolean=w466) -> (0, 1=w462:i16)
        n285 = Boolean To (0,1)(Boolean=w465) -> (0, 1=w464:i16)
        n286 = Negate(x=w464) -> (-x=w463:i16)
        n287 = Add(x=w462, y=w463) -> (x+y=w461:i16)
        n288 = call <vilib>:"NT Write Number.vi"("Numeric"=w461, "Name"=w460) -> ()  [unwired: 9 in, 1 out]
      }
      event "Ring": Value Change {
        n289 = event-data() -> ("NewVal"=w470:u16)  [unwired: 1 in]
        n290 = property on="Ring" class="Ring (strict)"() -> ("Strings []"=w471:string[])  [unwired: 2 in, 2 out]
        n291 = Index Array(array=w471, index=w470) -> (element=w469:string)
        n292 = call <vilib>:"NT Write String.vi"("String"=w469, "Name"=w468) -> ()  [unwired: 9 in, 1 out]
      }
    }
  }
  n293 = Index Array(array=w17) -> (element=w18:cluster{string[]})  [unwired: 1 in]
  n294 = Unbundle(w18) -> (w16:string[])
  n295 = Match First String(2:w16, 3:w15) -> (0:w14:i32)  [unwired: 1 out]
  n296 = Bundle("value"=w20, "value"=w19, "index"=w14) -> (w8:cluster{"value":i32, "value":i32, "index":i32})  [unwired: 1 out]
  n297 = property on="On/Off" class="Bool (strict)"("Visible"=w31) -> ()  [unwired: 2 in, 2 out]
  n298 = property on="Motor" class="Clust (strict)"("Visible"=w31) -> ()  [unwired: 2 in, 2 out]
  n299 = property on="Progress" class="Clust (strict)"("Visible"=w31) -> ()  [unwired: 2 in, 2 out]
  n300 = property on="Ring" class="Ring (strict)"("Visible"=w31) -> ()  [unwired: 2 in, 2 out]
  n301 = property on="Camera Settings" class="Clust (strict)"("Val(Sgnl)"=w8) -> ()  [unwired: 2 in, 2 out]
  n302 = property on="Rev/Fwd" class="Clust (strict)"("Visible"=w31) -> ()  [unwired: 2 in, 2 out]
  n303 = property on="Camera Settings" class="Clust (strict)"("Visible"=w31) -> ()  [unwired: 2 in, 2 out]
  n304 = local write "DB Camera Config"(w31) -> ()
  "Dashboard Code Verzion" <- "Vision Dash 1.1 Final" ("Dashboard Code Verzion")
